vi "3.3.vi"(0 "偏移量(0)":i32, 1 "长度（剩余）":i32, 2 "字符串":string, 3 "偏移量(0) 2":i32, 4 "长度（剩余） 2":i32, 5 "偏移量(0) 3":i32, 6 "长度（剩余） 3":i32) -> (7 "输出 1":dbl, 8 "子字符串":string, 9 "子字符串 2":string)   [LabVIEW 2017]
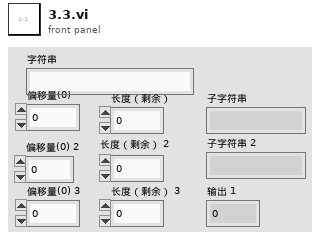
[diagram p1: front panel]
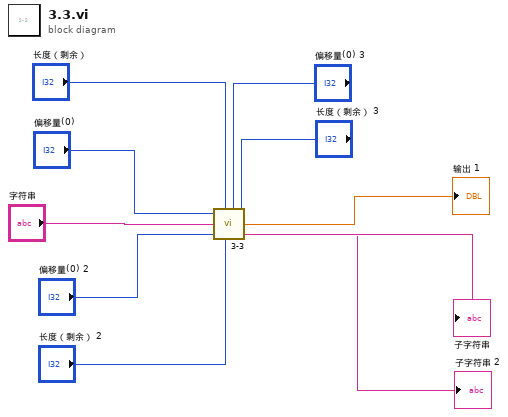
[diagram p0: block diagram]
diagram:
  n1 = call "3-3.vi"("偏移量(0)"="偏移量(0)", "长度（剩余）"="长度（剩余）", "字符串"="字符串", "偏移量(0) 2"="偏移量(0) 2", "长度（剩余） 2"="长度（剩余） 2", "偏移量(0) 3"="偏移量(0) 3", "长度（剩余） 3"="长度（剩余） 3") -> ("输出 1"=→"输出 1":dbl, "子字符串"=→"子字符串":string, "子字符串 2"=→"子字符串 2":string)
